vi "RDB Database.vi"(7 "Filter Cluster":string, 8 "error in (no error)":errorcluster, 11 "reference in":refnum<vi>) -> (0 "error out":errorcluster, 3 "reference out":refnum<vi>)   [LabVIEW 2023, in "Vires VTD System Explorer.lvlib"]
uses:
  System Explorer/Vires VTD System Explorer.lvlib
  <vilib>/xnet/xnet.llb/XNET String To IO Name (Database Alias).vi
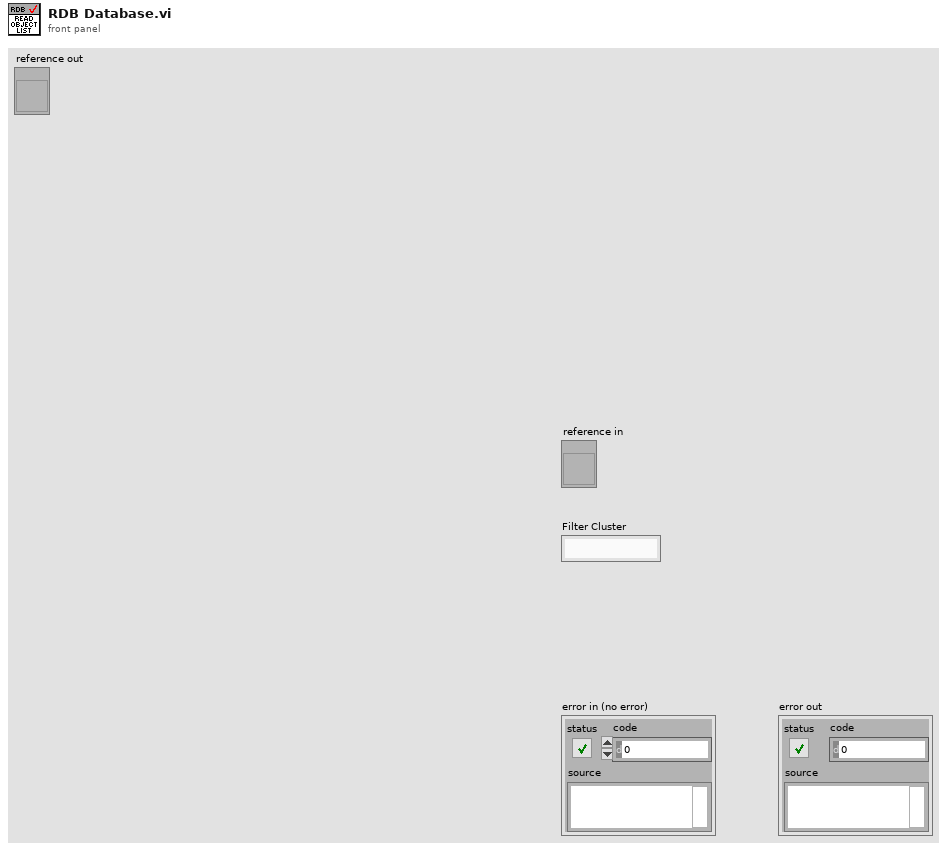
[diagram p1: front panel]
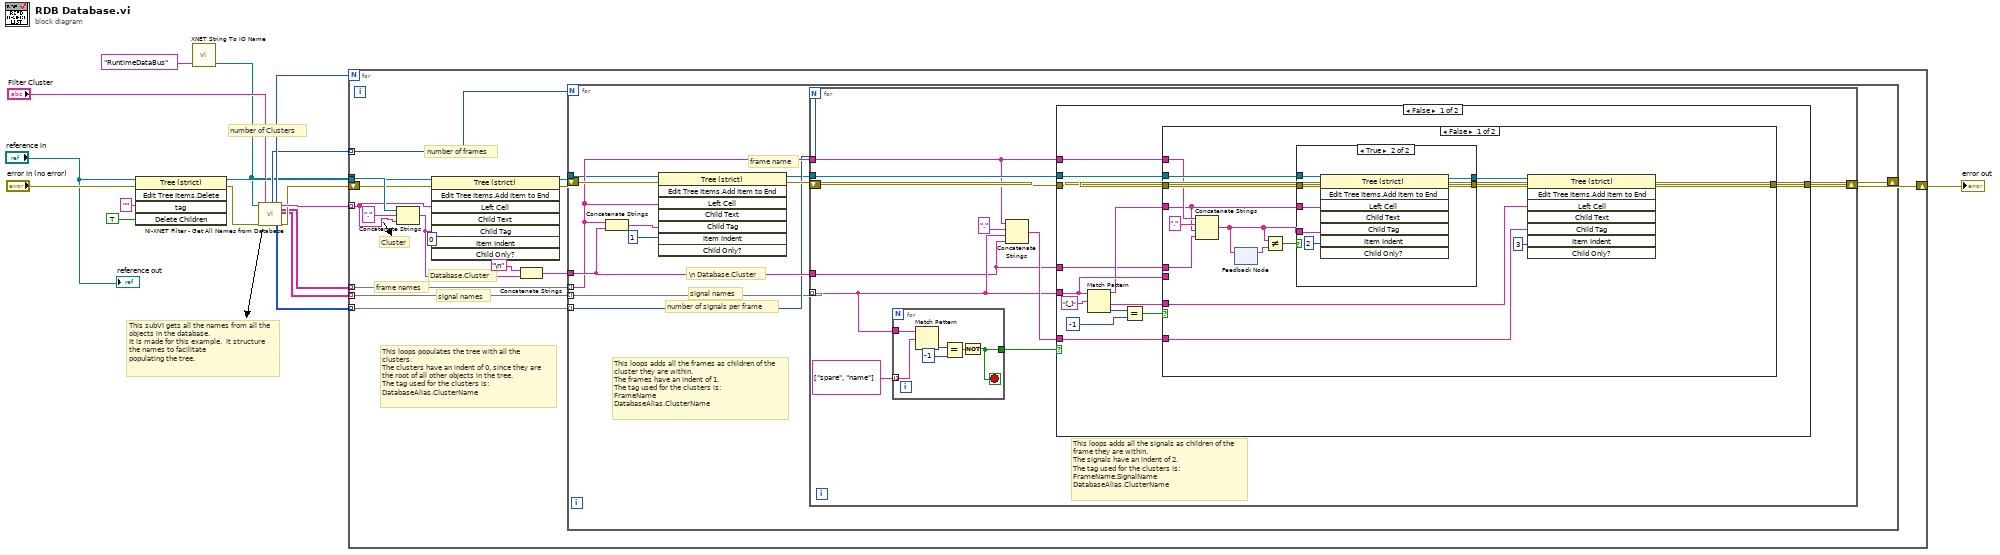
[diagram p0: block diagram]
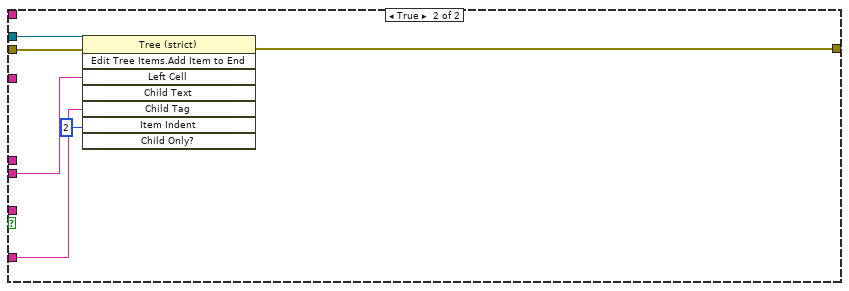
[diagram p3: hidden frame]
diagram:
  # "number of Clusters"
  # "This subVI gets all the names from all the objects in the database.\nIt is made for this example.  It structure the names to facilitate\npopulating the tree."
  n1 = invoke on="Invoke Node" class="Tree (strict)" method="Edit Tree Items.Delete"(reference="reference in", error in="error in (no error)", "tag"="" ("Tag"), "Delete Children"=TRUE ("Delete Children?")) -> (reference out=w6:refnum<vi>, error out=w2:errorcluster)  [unwired: 1 in, 3 out]
  n2 = call-poly <vilib>:"XNET String To IO Name.vi"("string"="RuntimeDataBus" ("element")) -> ("XNET Database"=w3:refnum<k21>)  [unwired: 4 out]
  n3 = call "NI-XNET Filter - Get All Names from Database.vi"("database in (:memory:)"=w3, "error in (no error)"=w2, "Filter Cluster"="Filter Cluster") -> ("Number of Frames"=w10:i32[], "Number of Clusters"=w13:i32, "Number of Signals"=w9:i32[][], "Clusters"=w15:string[], "Frames"=w11:string[][], "Signals"=w8:string[][][], "error out"=w14:errorcluster)  [unwired: 10 in]
  n4 = for {
    N: w13 -> [_]
    tunnel: w15 -> [w28] mode=indexing
    tunnel: w11 -> [w22] mode=indexing
    tunnel: w10 -> [w31] mode=indexing
    tunnel: w3 -> [w29]
    tunnel: w9 -> [w21] mode=indexing
    tunnel: w8 -> [w20] mode=indexing
    shift-right: [w32] -> w12
    shift-left: w14 -> [w24]
    tunnel: w6 -> [w19]
    # "Cluster"
    # "Database.Cluster"
    # "number of frames"
    # "signal names"
    # "frame names"
    # "This loops populates the tree with all the clusters.\nThe clusters have an indent of 0, since they are the root of all other objects in the tree.\nThe tag used for the clusters is: \nDatabaseAlias.ClusterName"
    n5 = Concatenate Strings(w29, "." ("string"), w28) -> (w26:string)
    n6 = invoke on="Invoke Node" class="Tree (strict)" method="Edit Tree Items.Add Item to End"(reference=w19, error in=w24, "Left Cell"=w28, "Child Tag"=w26, "Item Indent"=0 ("New Item Indentation")) -> (reference out=w18:refnum<vi>, error out=w33:errorcluster)  [unwired: 3 in, 6 out]
    n7 = Concatenate Strings("\n", w26) -> (w25:string)
    n8 = for {
      N: w31 -> [_]
      tunnel: w22 -> [w38] mode=indexing
      tunnel: w25 -> [w40]
      tunnel: w21 -> [w37] mode=indexing
      tunnel: w20 -> [w36] mode=indexing
      shift-right: [w43] -> w32
      shift-left: w33 -> [w42]
      tunnel: w18 -> [w35]
      # "\\n Database.Cluster"
      # "signal names"
      # "number of signals per frame"
      # "frame name"
      # "This loops adds all the frames as children of the cluster they are within.\nThe frames have an indent of 1.\nThe tag used for the clusters is: \nFrameName\nDatabaseAlias.ClusterName"
      n9 = Concatenate Strings(w38, w40) -> (w39:string)
      n10 = invoke on="Invoke Node" class="Tree (strict)" method="Edit Tree Items.Add Item to End"(reference=w35, error in=w42, "Left Cell"=w38, "Child Tag"=w39, "Item Indent"=1 ("New Item Indentation")) -> (reference out=w34:refnum<vi>, error out=w41:errorcluster)  [unwired: 3 in, 6 out]
      n11 = for {
        N: w37 -> [_]
        tunnel: w40 -> [w45]
        tunnel: w38 -> [w46]
        tunnel: w36 -> [w50] mode=indexing
        shift-right: [w54] -> w43
        shift-left: w41 -> [w53]
        tunnel: w34 -> [w47]
        # "This loops adds all the signals as children of the frame they are within.\nThe signals have an indent of 2.\nThe tag used for the clusters is: \nFrameName.SignalName\nDatabaseAlias.ClusterName"
        n12 = for {
          tunnel: w50 -> [w104]
          tunnel: string[] ["spare", "name"] -> [w103] mode=indexing
          tunnel: [w99] -> w48
          stop <- w99 stop-if-true
          n13 = Match Pattern(string=w104, regular expression=w103) -> (offset past match=w102:i32)  [unwired: 1 in, 3 out]
          n14 = Equal?(x=w102, y=-1) -> (x = y?=w100:bool)
          n15 = Not(x=w100) -> (.not. x?=w99:bool)
        }
        n16 = Concatenate Strings(w46, "." ("string"), w50, w45) -> (w52:string)
        n17 = case shown="False" w48 {
          tunnel: [w65 w98] -> w54
          tunnel: w53 -> [w67 w98]
          tunnel: w52 -> [w64 _]
          tunnel: w50 -> [w59 _]
          tunnel: w47 -> [w66 _]
          tunnel: w46 -> [w56 _]
          tunnel: w45 -> [w55 _]
          frame False {
            n18 = Match Pattern(string=w59, regular expression="[_]") -> (before substring=w58:string, after substring=w57:string, offset past match=w61:i32)  [unwired: 1 in, 1 out]
            n19 = Equal?(x=w61, y=-1) -> (x = y?=w60:bool)
            n20 = case shown="False" w60 {
              tunnel: w67 -> [w82 w97]
              tunnel: w66 -> [w81 w96]
              tunnel: [w78 w92] -> w65
              tunnel: w64 -> [w77 w94]
              tunnel: w59 -> [_ w93]
              tunnel: w58 -> [w72 _]
              tunnel: w57 -> [w75 _]
              tunnel: w56 -> [w74 _]
              tunnel: w55 -> [w71 _]
              frame False {
                n21 = Concatenate Strings(w74, "." ("string"), w72, w71) -> (w69:string)
                n22 = feedback-in #1(w69) -> ()
                n23 = feedback #1() -> (w70:string)  [unwired: 1 in]
                n24 = Not Equal?(x=w69, y=w70) -> (x != y?=w68:bool)
                n25 = case shown="True" w68 {
                  tunnel: w82 -> [w83 w91]
                  tunnel: w81 -> [w84 w90]
                  tunnel: [w84 w88] -> w80
                  tunnel: [w83 w87] -> w79
                  tunnel: w72 -> [_ w86]
                  tunnel: w69 -> [_ w85]
                  frame False {
                  }
                  frame True {
                    n26 = invoke on="Invoke Node" class="Tree (strict)" method="Edit Tree Items.Add Item to End"(reference=w90, error in=w91, "Left Cell"=w86, "Child Tag"=w85, "Item Indent"=2 ("New Item Indentation")) -> (reference out=w88:refnum<vi>, error out=w87:errorcluster)  [unwired: 3 in, 6 out]
                  }
                }
                n27 = invoke on="Invoke Node" class="Tree (strict)" method="Edit Tree Items.Add Item to End"(reference=w80, error in=w79, "Left Cell"=w75, "Child Tag"=w77, "Item Indent"=3 ("New Item Indentation")) -> (error out=w78:errorcluster)  [unwired: 3 in, 7 out]
              }
              frame True {
                n28 = invoke on="Invoke Node" class="Tree (strict)" method="Edit Tree Items.Add Item to End"(reference=w96, error in=w97, "Left Cell"=w93, "Child Tag"=w94, "Item Indent"=2 ("New Item Indentation")) -> (error out=w92:errorcluster)  [unwired: 3 in, 7 out]
              }
            }
          }
          frame True {
          }
        }
      }
    }
  }
  "error out" <- w12
  "reference out" <- "reference in"
